vi "Write Battery Data.vi"(8 "error in (no error)":errorcluster, 10 "Battery Pack Info":T1, 11 "Battery Message in":refnum<class "Battery Message.lvclass">) -> (0 "error out":errorcluster, 3 "Battery Message out":refnum<class "Battery Message.lvclass">)   [LabVIEW 2015, in "RDS Child Messages.lvlib" / "Battery Message.lvclass"]
uses:
  Battery Message.lvclass
  RDS Instruments/Battery/Battery Data.ctl
  Battery Status.ctl
  Battery Message.lvclass/Battery Message.ctl
  RDS Instruments/RDS Instrument Library.lvlib
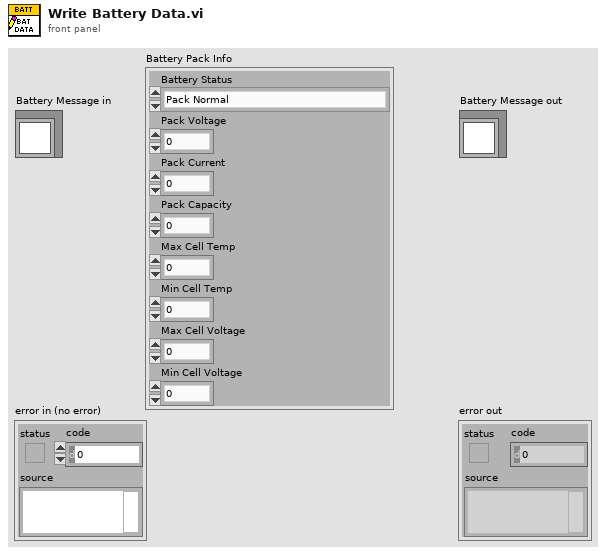
[diagram p1: front panel]
types:
  T1 = typedef "RDS Instrument Library.lvlib/Battery Data.ctl" = cluster{"Battery Status":T2, "Pack Voltage":sgl, "Pack Current":sgl, "Pack Capacity":sgl, "Max Cell Temp":sgl, "Min Cell Temp":sgl, "Max Cell Voltage":sgl, "Min Cell Voltage":sgl}
  T2 = typedef "RDS Instrument Library.lvlib/Battery Status.ctl" = enum16{"Pack Normal", "Alarm: Cell temp too high", "Alarm: Pack voltage too high", "Warn: Pack voltage too high ", "Alarm: Pack voltage too low", "Warn: Pack voltage low", "Alarm Pack current too high", "Warn: Pack current too high ", "Fault: Pack to chassis connection detected", "Fault: Pack to cell connection error", "Fautl: System error"}
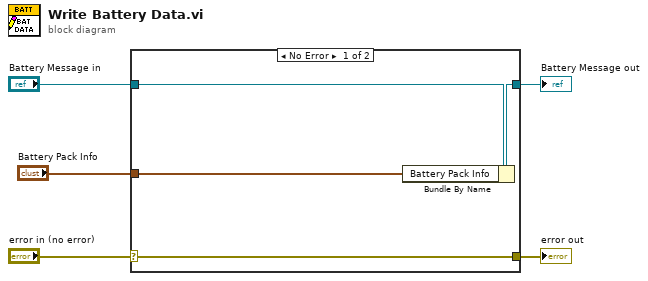
[diagram p0: block diagram]
diagram:
  n1 = case shown="No Error" "error in (no error)" {
    selector: "error in (no error)" -> [w9 w10]
    tunnel: [w9 w10] -> w4
    tunnel: [w7 w11] -> w2
    tunnel: "Battery Message in" -> [w8 w11]
    tunnel: "Battery Pack Info" -> [w6 _]
    frame No Error {
      n2 = Bundle By Name(cluster=w8, "Battery Pack Info"=w6) -> (w7:refnum<class "Battery Message.lvclass">)
    }
    frame Error {
    }
  }
  "error out" <- w4
  "Battery Message out" <- w2
